vi "Fields Marked as Indexed.vi"(7 "Fields In":T2[](array[typedef]), 8 "error in (no error)":errorcluster, 11 "Connection Refnum":T1) -> (0 "error out":errorcluster, 3 "Connection Refnum":T1, 5 "Fields Out":T2[](array[typedef]))   [LabVIEW 2011]
uses:
  Field Record.ctl
  Field DataTypes.ctl
  Field NextItem.ctl
  Summitek EXT/ODBC/SQL Controls/Connection Refnum.ctl
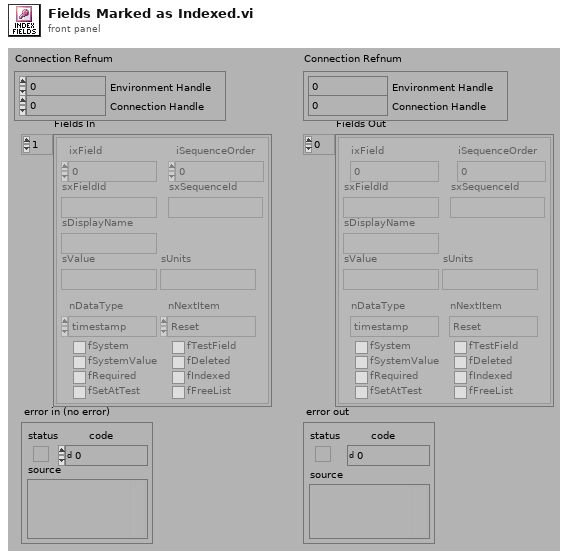
[diagram p1: front panel]
types:
  T1 = typedef "Connection Refnum.ctl" = cluster{"Environment Handle":i32, "Connection Handle":i32}
  T2 = typedef "Field Record.ctl" = cluster{"ixField":i32, "iSequenceOrder":i32, "sxFieldId":string, "sxSequenceId":string, "sDisplayName":string, "sValue":string, "sUnits":string, "nDataType":T3, "nNextItem":T4, "fSystem":bool, "fSystemValue":bool, "fRequired":bool, "fSetAtTest":bool, "fTestField":bool, "fDeleted":bool, "fIndexed":bool, "fFreeList":bool}
  T3 = typedef "Field DataTypes.ctl" = enum32{"text", "numeric", "list", "timestamp", "boolean"}
  T4 = typedef "Field NextItem.ctl" = enum32{"Reset", "Retain", "Auto-Increment"}
  T5 = typedef "Statement Refnum.ctl" = cluster{"Statement Handle":i32, "Parameter Number":u16}
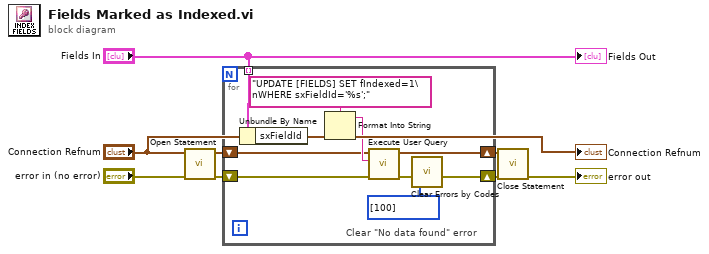
[diagram p0: block diagram]
diagram:
  n1 = call "Open Statement.vi"("error in (no error)"="error in (no error)", "Connection Refnum"="Connection Refnum") -> ("error out"=w8:errorcluster, "Statement Refnum"=w5:T5)  [unwired: 4 out]
  n2 = for {
    shift-right: [w15] -> w7
    shift-left: w8 -> [w14]
    shift-right: [w12] -> w6
    shift-left: w5 -> [w11]
    tunnel: "Fields In" -> [w10] mode=indexing
    # "Clear \"No data found\" error"
    n3 = Unbundle By Name(w10) -> ("sxFieldId"=w18:string)
    n4 = Format Into String(format string="UPDATE [FIELDS] SET fIndexed=1\nWHERE sxFieldId='%s';" ("User Query"), w18) -> (resulting string=w16:string)  [unwired: 2 in, 1 out]
    n5 = call "Execute User Query.vi"("error in (no error)"=w14, "User Query"=w16, "Statement Refnum"=w11) -> ("error out"=w13:errorcluster, "Statement Refnum"=w12:T5)  [unwired: 1 in, 2 out]
    n6 = call "Clear Errors by Codes.vi"("Error Codes\nto Clear (Empty)"=i32[] [100] ("Error Codes\nto Clear (Empty)"), "error in (no error)"=w13) -> ("error out"=w15:errorcluster)  [unwired: 5 out]
  }
  n7 = call "Close Statement.vi"("error in (no error)"=w7, "Statement Refnum"=w6) -> ("error out"=→"error out":errorcluster)  [unwired: 5 out]
  "Fields Out" <- "Fields In"
  "Connection Refnum" <- "Connection Refnum"
